vi "concentration.vi"(8 "error in":errorcluster, 9 "List ROI in":dbl[][](array[numeric]), 10 "List Concentration":T2(array[cluster]) {"N. Peak" items=["0.000000", "1.000000", "2.000000", "3.000000", "4.000000", "5.000000", "6.000000", "7.000000", "8.000000", "9.000000", "10.000000", "11.000000"]}, 11 "Elements Selected":string[][](table)) -> (0 "error out":errorcluster, 3 "Concentration":T1)   [LabVIEW 2023]
uses:
  control/Concentrations.ctl
  control/global name path.vi
  python_to_labview/global python version.vi
  <vilib>/Utility/file.llb/Write Delimited Spreadsheet (string).vi
  <vilib>/Utility/file.llb/Read Delimited Spreadsheet (string).vi
  queue/Front Panel Message Queue.lvlib
panel:
  out "Parameters\nready":bool
  out "Loading":bool
  in  "Type Conentration":enum32{"Item 0", "Item 1"}(radio)
  in  "Load File":path
  in  "load":bool
  in  "save":bool
  out "XY Graph":cluster{"Z":i32[], "Param":dbl[]}[](graph)
  in  "conc":bool
  in  "setup":bool
  in  "Stop":bool
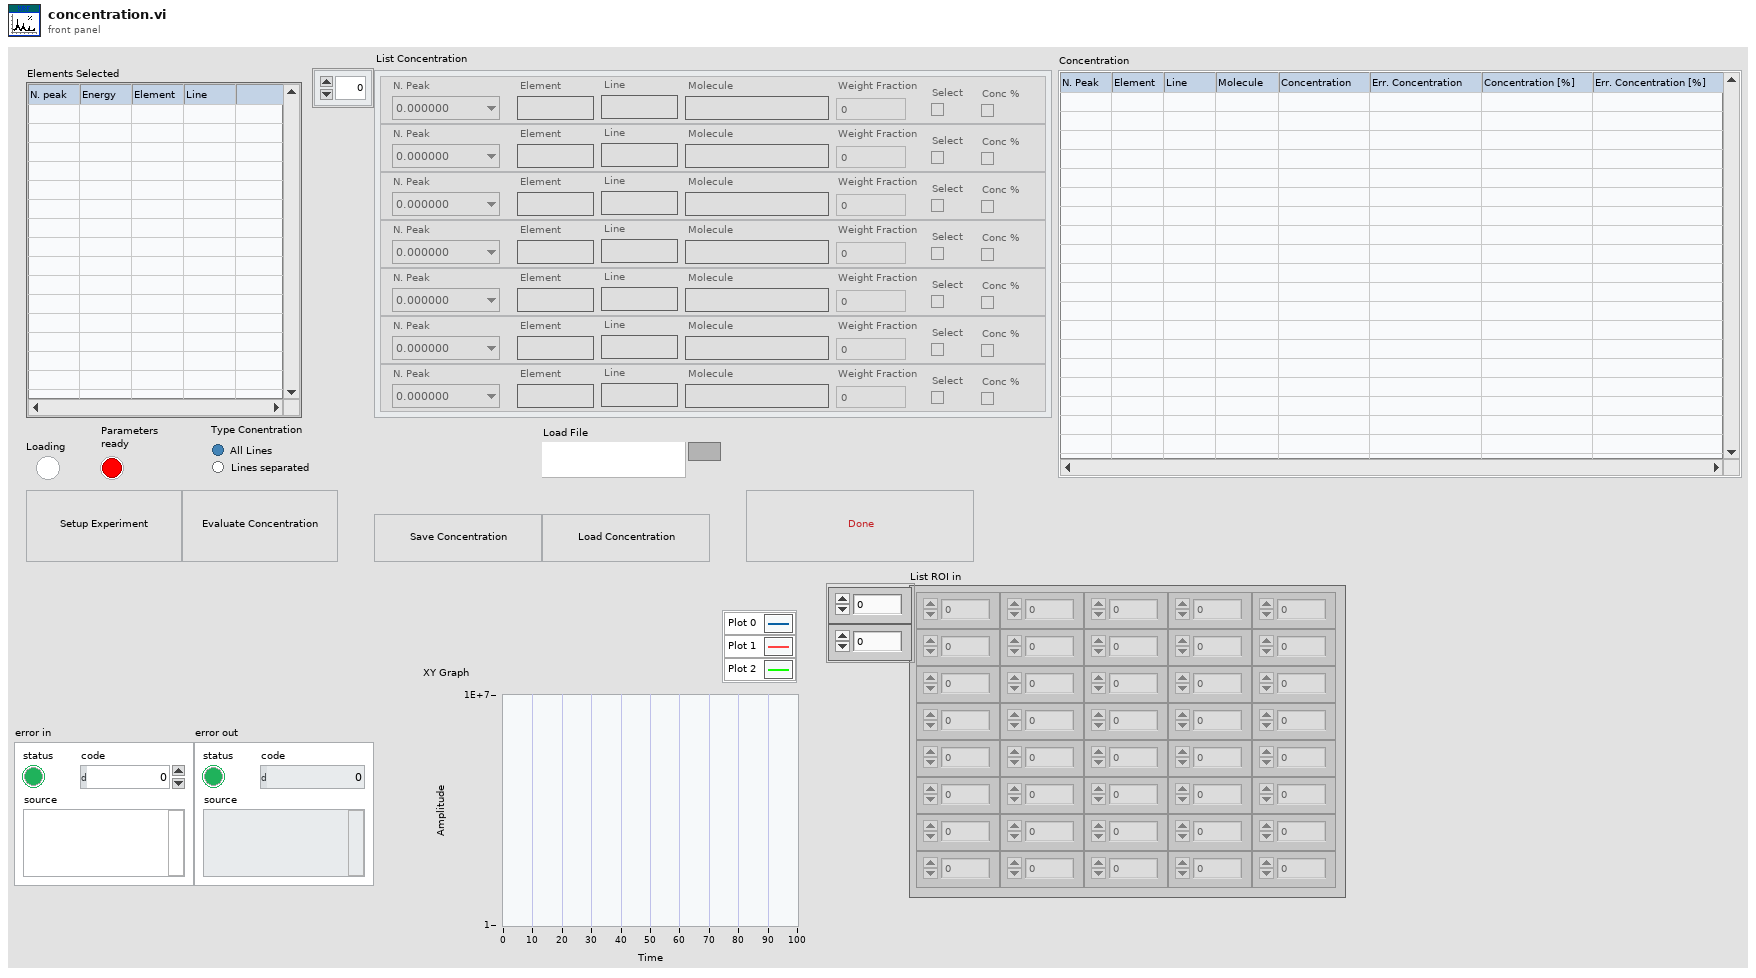
[diagram p1: front panel]
types:
  T1 = typedef "Concentrations.ctl" = string[][]
  T2 = cluster{"N. Peak":u16, "Element":string, "Molecule":string, "Weight Fraction":dbl, "Select":bool, "Conc %":bool, "Line":string}[]
  T3 = typedef "Front Panel Message Queue.lvlib/load Message Queues.ctl" = cluster{"Main":refnum<queue>}
  T4 = cluster{"N. Peak":u16, "Element":string, "Molecule":string, "Weight Fraction":dbl, "Select":bool, "Conc %":bool, "Line":string}
  T5 = cluster{"source-Kalpha":dbl[][], "source-Kbeta":dbl[][], "source-Lalpha":dbl[][]}
  T6 = cluster{"detector-Kalpha":dbl[][], "detector-Kbeta":dbl[][], "detector-Lalpha":dbl[][]}
  T7 = typedef "Parameters.ctl" = cluster{"Z":i32[], "Param":dbl[]}
  T8 = cluster{"N. Peak":u16, "Element":string, "Molecule":string, "Weight Fraction":dbl, "Select":bool, "Conc %":bool}[]
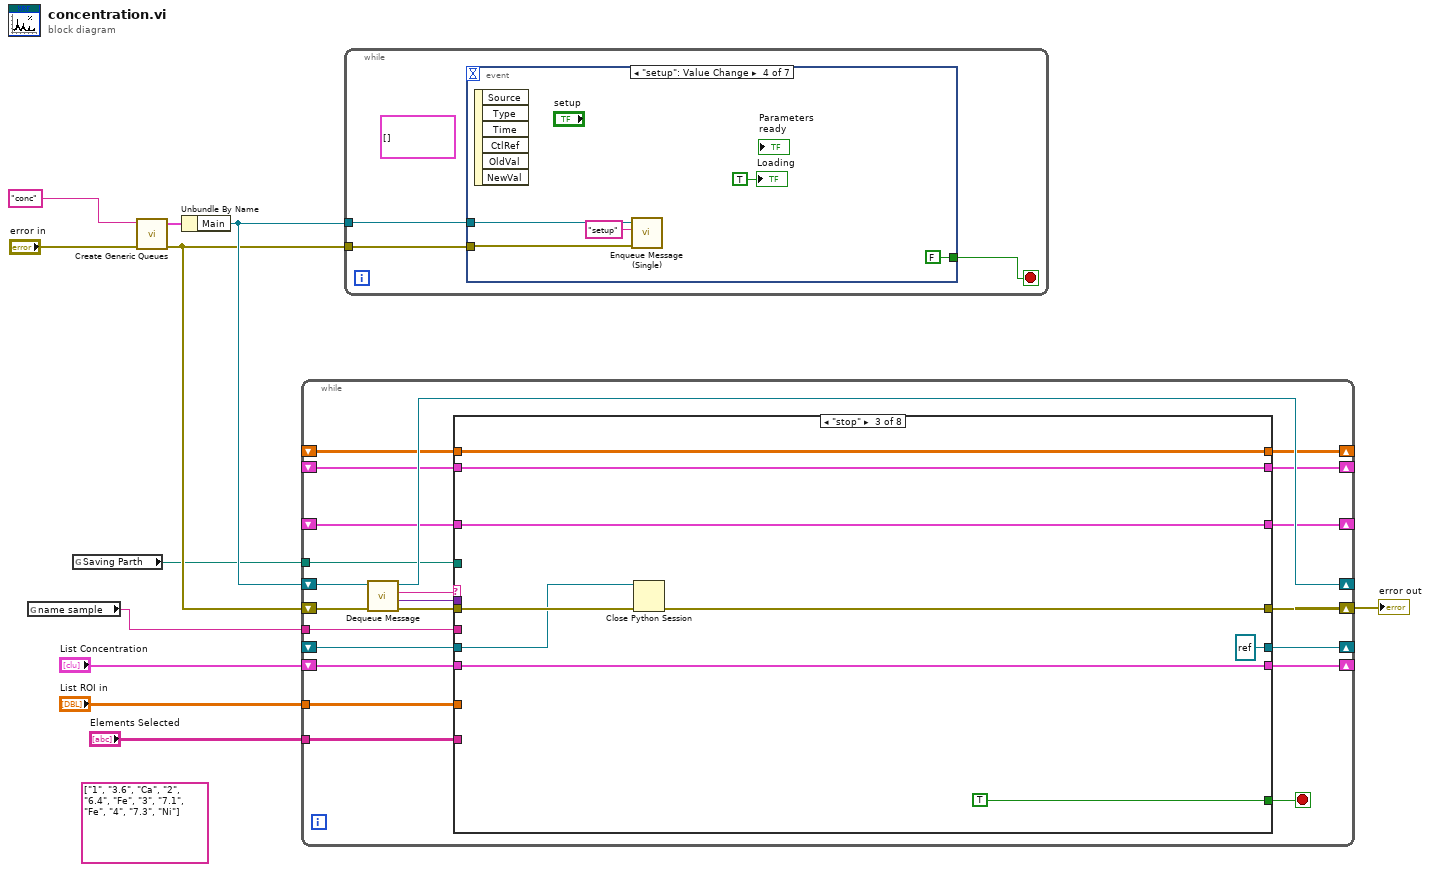
[diagram p0: block diagram]
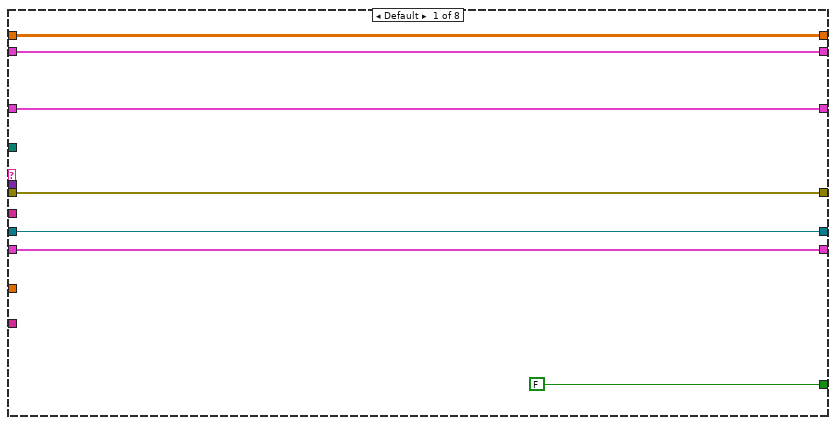
[diagram p2: hidden frame]
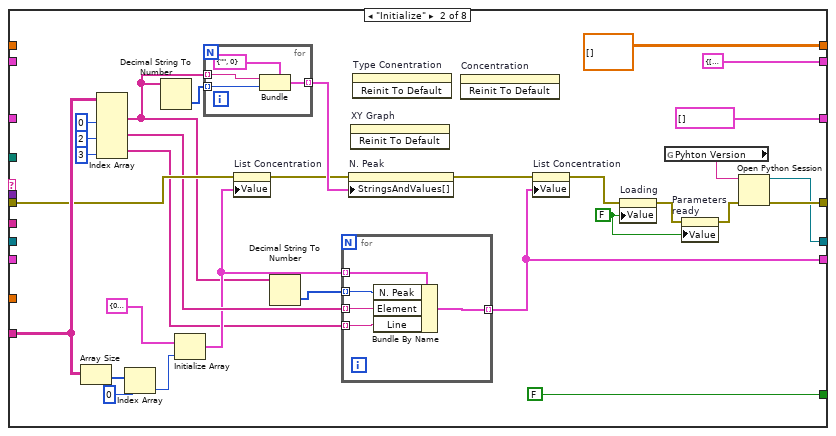
[diagram p3: hidden frame]
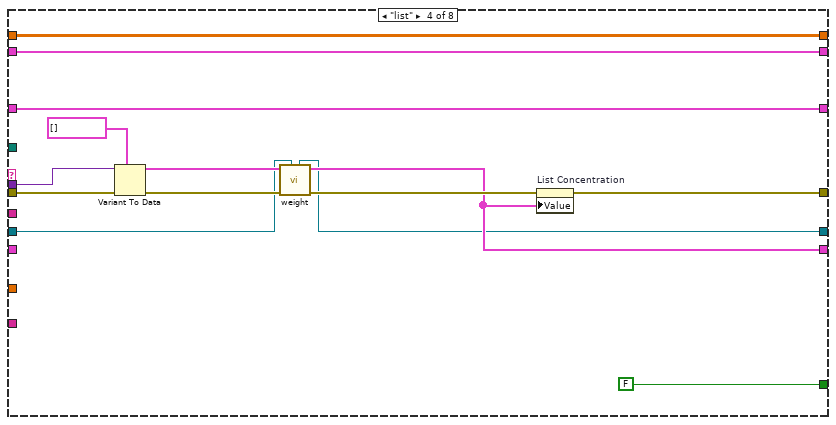
[diagram p4: hidden frame]
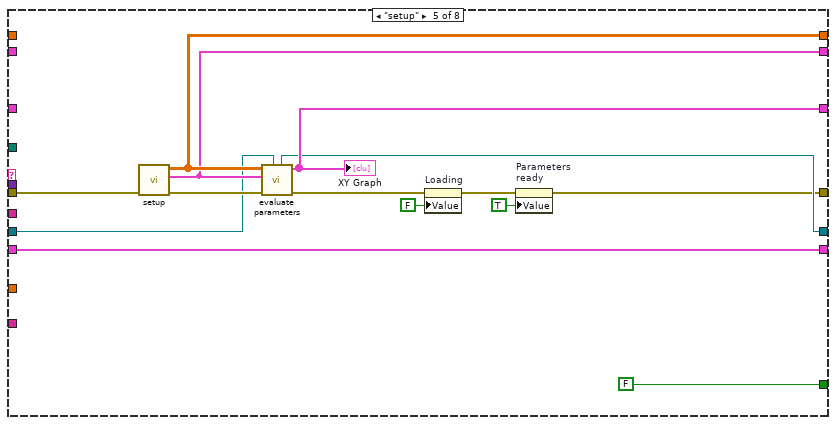
[diagram p5: hidden frame]
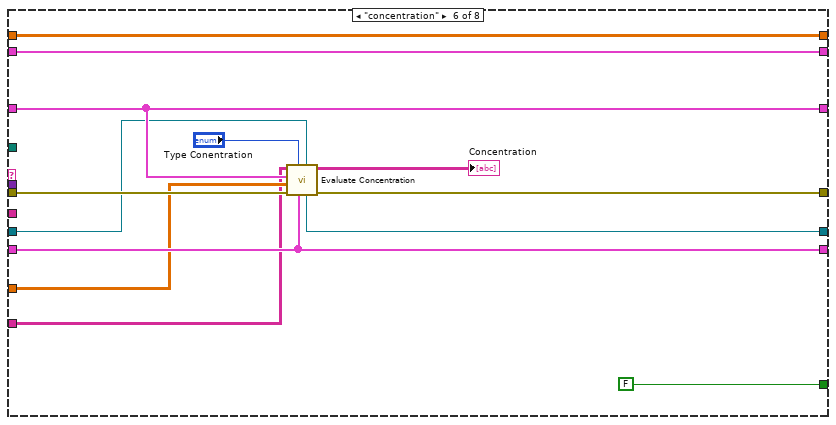
[diagram p6: hidden frame]
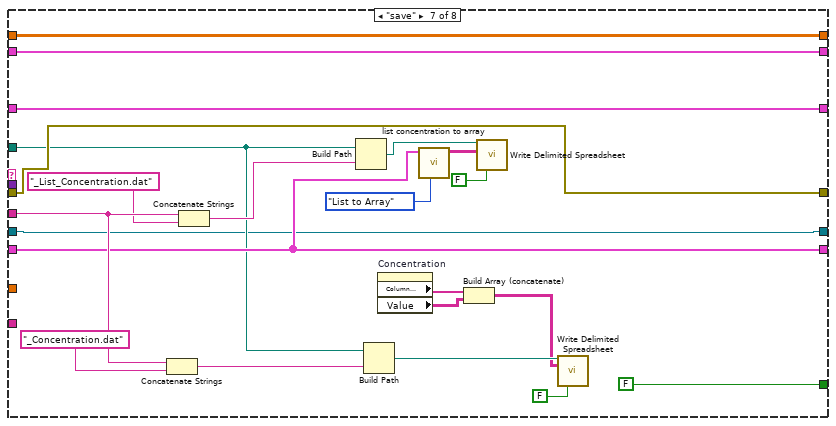
[diagram p7: hidden frame]
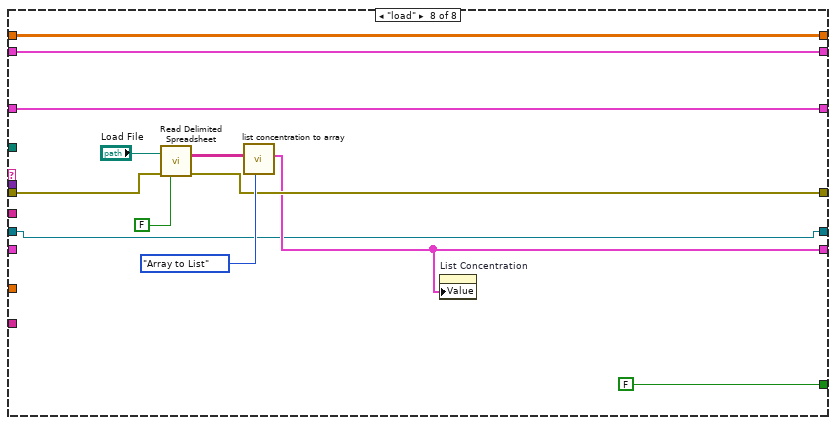
[diagram p8: hidden frame]
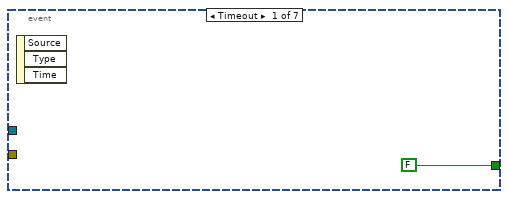
[diagram p9: hidden frame]
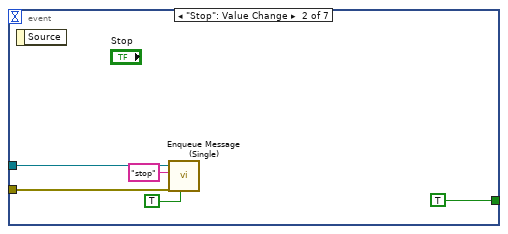
[diagram p10: hidden frame]
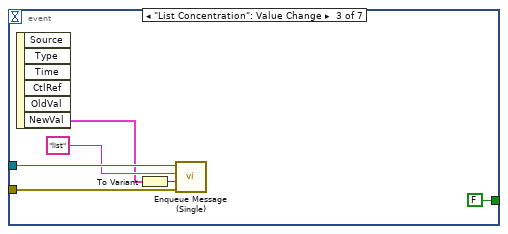
[diagram p11: hidden frame]
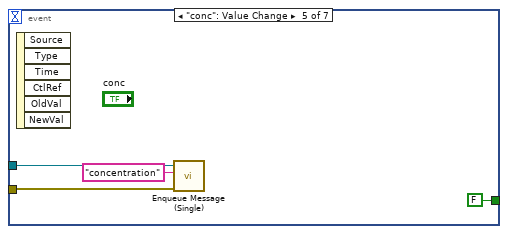
[diagram p12: hidden frame]
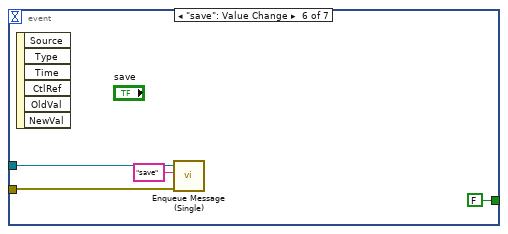
[diagram p13: hidden frame]
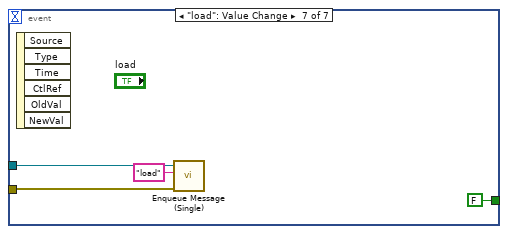
[diagram p14: hidden frame]
diagram:
  (unwired) string[][] [["1", "3.6", "Ca"], ["2", "6.4", "Fe"], ["3", "7.1", "Fe"], ["4", "7.3", "Ni"]] ("Elements Selected")
  n1 = global read "global name path.vi" "name sample"() -> (w1:string)
  n2 = global read "global name path.vi" "Saving Parth"() -> (w2:path)
  n3 = call "Create Generic Queues.vi"("error in (no error)"="error in", "name"="conc") -> ("error out"=w6:errorcluster, "Message Queues"=w8:T3)  [unwired: 8 in]
  n4 = Unbundle By Name(w8) -> ("Main"=w7:refnum<queue>)
  n5 = while {
    tunnel: "List ROI in" -> [w26]
    tunnel: "Elements Selected" -> [w25]
    shift-right: [w28] -> w5
    shift-left: w6 -> [w32]
    shift-right: [w31] -> _
    shift-left: w7 -> [w33]
    shift-right: [w24] -> _
    shift-left: "List Concentration" -> [w23]
    shift-right: [w21] -> _
    shift-left: _ -> [w19]
    shift-right: [w20] -> _
    shift-left: _ -> [w18]
    shift-right: [w17] -> _
    shift-left: _ -> [w16]
    tunnel: w1 -> [w15]
    tunnel: w2 -> [w14]
    shift-right: [w13] -> _
    shift-left: _ -> [w12]
    stop <- w27 stop-if-true
    n6 = call "Dequeue Message.vi"("error in (no error)"=w32, "Message Queue"=w33) -> ("error out"=w30:errorcluster, "Message Data"=w22:variant, "Message"=w29:string, "dup Message Queue"=w31:refnum<queue>)  [unwired: 5 in, 1 out]
    n7 = case shown="\"stop\"" w29 {
      tunnel: w30 -> [w40 w60 w83 w102 w114 w126 w140 w158]
      tunnel: [w40 w46 w82 w97 w104 w125 w140 w159] -> w28
      tunnel: [FALSE FALSE TRUE FALSE FALSE FALSE FALSE FALSE] -> w27
      tunnel: w26 -> [_ _ _ _ _ w122 _ _]
      tunnel: w25 -> [_ w63 _ _ _ w121 _ _]
      tunnel: [w38 w56 w87 w95 w115 w124 w141 w153] -> w24
      tunnel: w23 -> [w38 _ w87 _ w115 w124 w141 _]
      tunnel: w22 -> [_ _ _ w101 _ _ _ _]
      tunnel: [w37 dbl[][] [] ("Source Out") w86 w94 w113 w128 w139 w155] -> w21
      tunnel: [w36 T5 {"source-Kalpha"=[], "source-Kbeta"=[], "source-Lalpha"=[]} ("source-lines") w85 w93 w112 w127 w138 w156] -> w20
      tunnel: w19 -> [w37 _ w86 w94 _ w128 w139 w155]
      tunnel: w18 -> [w36 _ w85 w93 _ w127 w138 w156]
      tunnel: [w35 cluster{"Z":i32[], "Param":dbl[]}[] [] ("Experimental Parameters") w84 w92 w110 w123 w132 w157] -> w17
      tunnel: w16 -> [w35 _ w84 w92 _ w123 w132 w157]
      tunnel: w15 -> [_ _ _ _ _ _ w150 _]
      tunnel: w14 -> [_ _ _ _ _ _ w131 _]
      tunnel: [w34 w45 refnum<k35> refnum ("session out") w89 w109 w117 w130 w152] -> w13
      tunnel: w12 -> [w34 _ w80 w90 w108 w118 w130 w152]
      frame Default {
      }
      frame "Initialize" {
        w41 = FALSE ("Loading")
        n8 = Array Size(array=w63) -> (size(s)=w67:i32[])
        n9 = Index Array(array=w63, index (col) #1=0 ("disabled index (col)"), index (col) #2=2 ("index (col)"), index (col) #3=3 ("index (col)")) -> (element #1=w53:string[], element #2=w59:string[], element #3=w48:string[])  [unwired: 3 in]
        n10 = Index Array(array=w67, index=0) -> (element=w65:i32)
        n11 = Decimal String To Number(string=w53) -> (number=w64:i32[])  [unwired: 2 in, 1 out]
        n12 = Initialize Array(T4 {"N. Peak"=0, "Element"="", "Molecule"="", "Weight Fraction"=0.0, "Select"=FALSE, "Conc %"=FALSE, "Line"=""} ("conc"), w65) -> (w58:T2)
        n13 = for {
          tunnel: w64 -> [w78] mode=indexing
          tunnel: w53 -> [w77] mode=indexing
          tunnel: [w76] -> w62 mode=indexing
          n14 = Bundle(cluster=cluster{string, u16} {"", 0}, w77, w78) -> (w76:cluster{string, u16})
        }
        n15 = property on="List Concentration" class="Arr (strict)"(error in=w60, "Value"=w58) -> (error out=w61:errorcluster)  [unwired: 1 in, 1 out]
        n16 = Decimal String To Number(string=w53) -> (number=w54:i32[])  [unwired: 2 in, 1 out]
        n17 = for {
          tunnel: w58 -> [w75] mode=indexing
          tunnel: w59 -> [w74] mode=indexing
          tunnel: [w73] -> w56 mode=indexing
          tunnel: w54 -> [w72] mode=indexing
          tunnel: w48 -> [w71] mode=indexing
          n18 = Bundle By Name(cluster=w75, "N. Peak"=w72, "Element"=w74, "Line"=w71) -> (w73:T4)
        }
        n19 = property on="N. Peak" class="Ring (strict)"(error in=w61, "StringsAndValues[]"=w62) -> (error out=w57:errorcluster)  [unwired: 1 in, 1 out]
        n20 = invoke on="XY Graph" class="XYGraph (strict)" method="Reinit To Default"() -> ()  [unwired: 3 in, 3 out]
        n21 = invoke on="Type Conentration" class="RadioBtnsControl (strict)" method="Reinit To Default"() -> ()  [unwired: 3 in, 3 out]
        n22 = invoke on="Concentration" class="Tbl (strict)" method="Reinit To Default"() -> ()  [unwired: 3 in, 3 out]
        n23 = property on="List Concentration" class="Arr (strict)"(error in=w57, "Value"=w56) -> (error out=w44:errorcluster)  [unwired: 1 in, 1 out]
        n24 = property on="Loading" class="Bool (strict)"(error in=w44, "Value"=w41) -> (error out=w43:errorcluster)  [unwired: 1 in, 1 out]
        n25 = global read "global python version.vi" "Pyhton Version"() -> (w47:string)
        n26 = property on="Parameters\nready" class="Bool (strict)"(error in=w43, "Value"=w41) -> (error out=w42:errorcluster)  [unwired: 1 in, 1 out]
        n27 = Open Python Session(python version=w47, 3:w42) -> (session out=w45:refnum<k35>, error out=w46:errorcluster)  [unwired: 1 in]
      }
      frame "stop" {
        n28 = Close Python Session(session in=w80, error in=w83) -> (11:w82:errorcluster)
      }
      frame "list" {
        n29 = Variant To Data(error in=w102, type=T2 [] ("List Concentration"), Variant=w101) -> (data=w98:T2, error out=w99:errorcluster)
        n30 = call "weight.vi"("python in"=w90, "error in"=w99, "List Concentration In"=w98) -> ("error out"=w96:errorcluster, "List Concentration Out"=w95:T2, "python out"=w89:refnum<k35>)  [unwired: 6 in]
        n31 = property on="List Concentration" class="Arr (strict)"(error in=w96, "Value"=w95) -> (error out=w97:errorcluster)  [unwired: 1 in, 1 out]
      }
      frame "setup" {
        n32 = call "setup.vi"("error in"=w114) -> ("error out"=w111:errorcluster, "detector-lines"=w112:T6, "Source Out"=w113:dbl[][])  [unwired: 8 in]
        n33 = call "evaluate parameters.vi"("python in"=w108, "error in"=w111, "detector-lines"=w112, "Source In"=w113) -> ("error out"=w106:errorcluster, "Parameters Out"=w110:T7[], "python out"=w109:refnum<k35>)  [unwired: 5 in]
        "XY Graph" <- w110
        n34 = property on="Loading" class="Bool (strict)"(error in=w106, "Value"=FALSE ("Loading")) -> (error out=w105:errorcluster)  [unwired: 1 in, 1 out]
        n35 = property on="Parameters\nready" class="Bool (strict)"(error in=w105, "Value"=TRUE ("Parameters\nready")) -> (error out=w104:errorcluster)  [unwired: 1 in, 1 out]
      }
      frame "concentration" {
        n36 = call "Evaluate Concentration.vi"("python in"=w118, "List Concentration In"=w124, "Type Conentration"="Type Conentration", "error in"=w126, "List ROI in"=w122, "Parameters In"=w123, "Elements Selected"=w121) -> ("error out"=w125:errorcluster, "Concentration"=→"Concentration":T1, "python out"=w117:refnum<k35>)  [unwired: 2 in]
      }
      frame "save" {
        n37 = Concatenate Strings(w150, "_Concentration.dat" ("string")) -> (w146:string)
        n38 = Concatenate Strings(w150, "_List_Concentration.dat" ("string")) -> (w147:string)
        n39 = Build Path(base path=w131, name or relative path=w147) -> (appended path=w145:path)
        n40 = Build Path(base path=w131, name or relative path=w146) -> (appended path=w144:path)
        n41 = property on="Concentration" class="Tbl (strict)"() -> ("Column Headers[]"=w135:string[], "Value"=w134:T1)  [unwired: 2 in, 2 out]
        n42 = call "list concentration to array.vi"("Type"=enum16{"List to Array", "Array to List"}."List to Array" ("Enum"), "List Concentration In"=w141) -> ("List String Out"=w142:string[][])  [unwired: 8 in, 1 out]
        n43 = Build Array (concatenate)(w135, w134) -> (w133:T1)
        n44 = call-poly <vilib>:"Write Delimited Spreadsheet.vi"("file path (dialog if empty)"=w145, "2D data"=w142, "transpose? (no:F)"=FALSE) -> ()  [unwired: 11 in, 2 out]
        n45 = call-poly <vilib>:"Write Delimited Spreadsheet.vi"("file path (dialog if empty)"=w144, "2D data"=w133, "transpose? (no:F)"=FALSE) -> ()  [unwired: 11 in, 2 out]
      }
      frame "load" {
        n46 = call-poly <vilib>:"Read Delimited Spreadsheet.vi"("file path (dialog if empty)"="Load File", "error in (no error)"=w158, "transpose? (F)"=FALSE) -> ("all rows"=w160:string[][], "error out"=w159:errorcluster)  [unwired: 7 in, 4 out]
        n47 = call "list concentration to array.vi"("Type"=enum16{"List to Array", "Array to List"}."Array to List" ("Enum"), "List String In"=w160) -> ("List Concentration Out"=w153:T2)  [unwired: 8 in, 1 out]
        n48 = property on="List Concentration" class="Arr (strict)"("Value"=w153) -> ()  [unwired: 2 in, 2 out]
      }
    }
  }
  "error out" <- w5
  n49 = while {
    tunnel: w7 -> [w165]
    tunnel: w6 -> [w164]
    stop <- w166 stop-if-true
    (unwired) T8 [] ("List Concentration")
    n50 = event shown="[3] \"setup\": Value Change" {
      selector: _ -> [_ _ _ _ _ _ _]
      dyn-events: _ -> [_ _ _ _ _ _ _]
      timeout: _ -> [_ _ _ _ _ _ _]
      tunnel: [FALSE TRUE FALSE FALSE FALSE FALSE FALSE] -> w166
      tunnel: w165 -> [_ w170 w176 w183 w187 w191 w195]
      tunnel: w164 -> [_ w171 w177 w182 w186 w190 w194]
      event Timeout {
        n51 = event-data() -> ()  [unwired: 1 in, 3 out]
      }
      event "Stop": Value Change {
        n52 = event-data() -> ()  [unwired: 1 in, 1 out]
        n53 = call "Enqueue Message (Single).vi"("Priority Message? (F)"=TRUE, "error in (no error)"=w171, "Message"="stop", "Message Queue"=w170) -> ()  [unwired: 6 in, 2 out]
      }
      event "List Concentration": Value Change {
        n54 = event-data() -> ("NewVal"=w174:T2)  [unwired: 1 in, 5 out]
        n55 = To Variant(anything=w174) -> (Variant=w173:variant)
        n56 = call "Enqueue Message (Single).vi"("error in (no error)"=w177, "Message Data"=w173, "Message"="list", "Message Queue"=w176) -> ()  [unwired: 6 in, 2 out]
      }
      event "setup": Value Change {
        n57 = event-data() -> ()  [unwired: 1 in, 6 out]
        n58 = call "Enqueue Message (Single).vi"("error in (no error)"=w182, "Message"="setup", "Message Queue"=w183) -> ()  [unwired: 7 in, 2 out]
        "Loading" <- TRUE ("Loading")
      }
      event "conc": Value Change {
        n59 = event-data() -> ()  [unwired: 1 in, 6 out]
        n60 = call "Enqueue Message (Single).vi"("error in (no error)"=w186, "Message"="concentration", "Message Queue"=w187) -> ()  [unwired: 7 in, 2 out]
      }
      event "save": Value Change {
        n61 = event-data() -> ()  [unwired: 1 in, 6 out]
        n62 = call "Enqueue Message (Single).vi"("error in (no error)"=w190, "Message"="save", "Message Queue"=w191) -> ()  [unwired: 7 in, 2 out]
      }
      event "load": Value Change {
        n63 = event-data() -> ()  [unwired: 1 in, 6 out]
        n64 = call "Enqueue Message (Single).vi"("error in (no error)"=w194, "Message"="load", "Message Queue"=w195) -> ()  [unwired: 7 in, 2 out]
      }
    }
  }
